vi "readBSfile.vi"() -> ()   [LabVIEW 2015]
doc: "Created by Artem Shevelev\nLabVIEW Portal profile: http://www.labviewportal.org/memberlist.php?mode=viewprofile&u=2340\ne-mail: artem.sh@gmail.com\nshevelev.pro"
panel:
  out "string":string
  out "data":u8[](array[numeric]) format="%02x"
  # "1\n0"
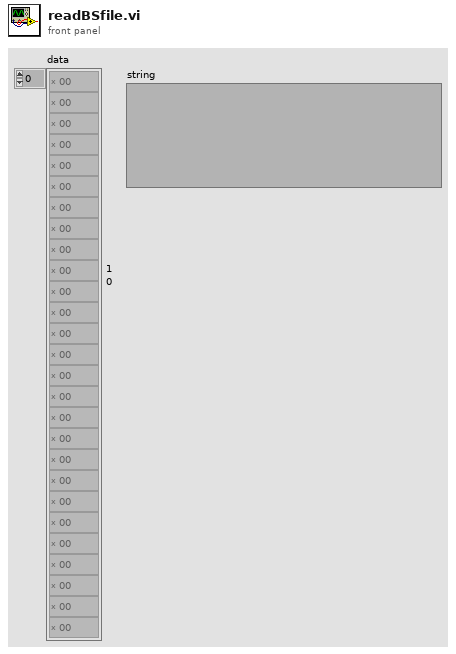
[diagram p1: front panel]
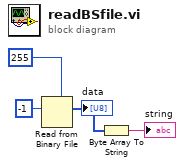
[diagram p0: block diagram]
diagram:
  n1 = Read from Binary File(5:u8 255, 10:-1 ("count (1)")) -> (2:w1:u8[])  [unwired: 4 in, 3 out]
  "data" <- w1
  n2 = Byte Array To String(unsigned byte array=w1) -> (string=→"string":string)
